vi "saveToTIFF.vi"(1 "Array":i32[][][](array[numeric]), 2 "selected path":path=path "C:/Users/Administrator/Desktop/tiff.tiff") -> ()   [LabVIEW 2016]
panel:
  out "max value 2":u16
  out "max value":u16
  out "Intensity Graph 2":u16[][](graph)
  in  "path to JPEG file":path=path "C:/Users/Administrator/Desktop/tiff.jpeg"
  out "Intensity Graph":u16[][](graph)
  in  "file path (use dialog)":path=path "C:/Users/Administrator/Desktop/binary.txt"
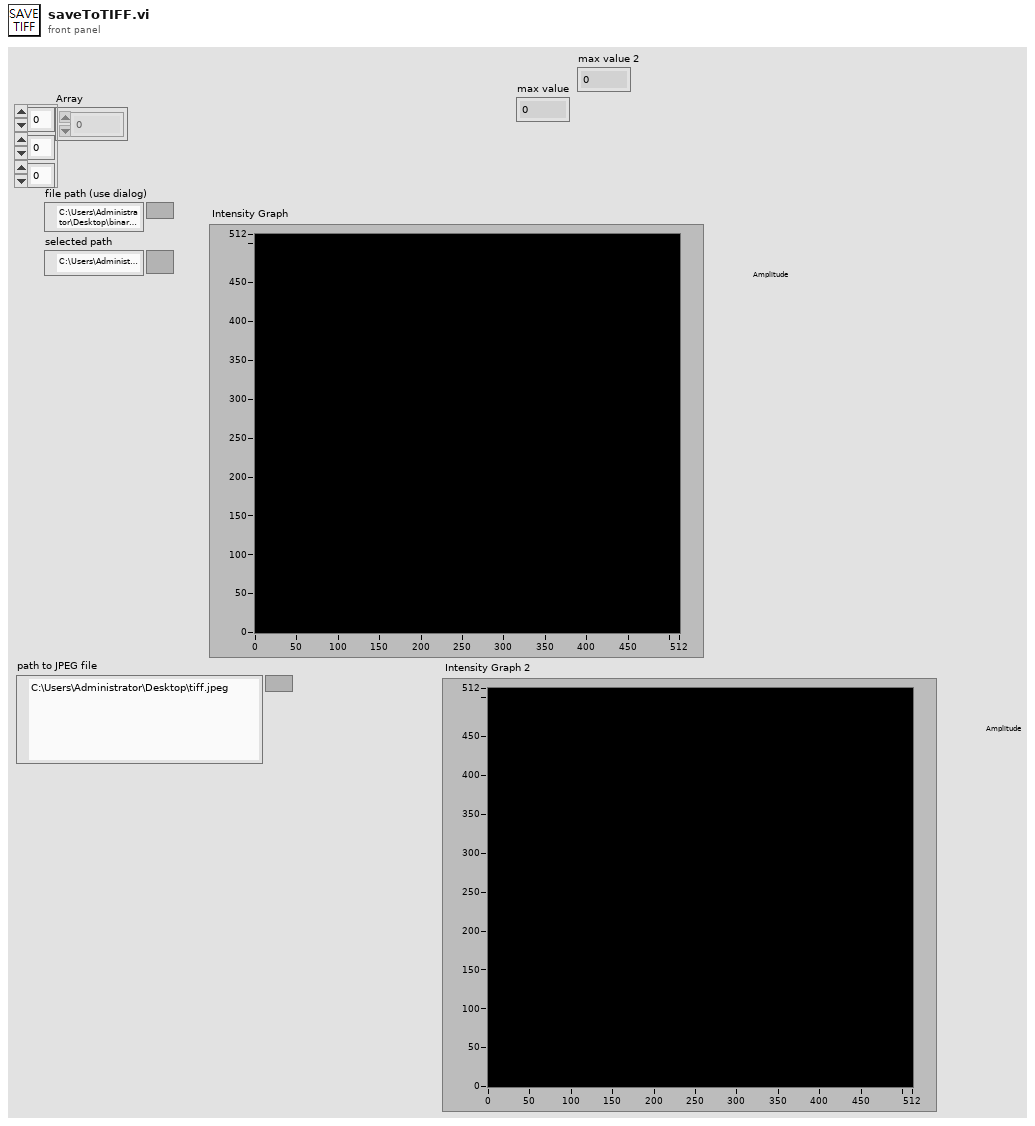
[diagram p1: front panel]
types:
  T1 = cluster{"SPEC":cluster{"CCD":cluster{"ModuleNo":string, "SerialNo":string, "CCD Type":string, "Counts":i32, "PixelNumber":i32, "PixelSize":dbl, "Exposure(ms )":dbl, "Average":i32, "Boxcar":i32, "binFactor":i32, "Reversion":bool, "Andor":cluster{"Temp. Target":i32, "Temp Stablized?":bool, "Readout List":string[], "RreAmp List":string[], "VSS List":string[], "Readout":u16, "PreAmp":u16, "VSS":u16, "Temp. Min":i32, "Temp. Max":i32, "OutputAmp List":string[], "OutputAmp":u16}, "Kinetic No":i32, "AccumCT":dbl, "KineticCT":dbl, "AcqMode":enum16{"Monitor", "Acquisition"}, "SpectraProcess":enum16{"Absorption", "TakeRef", "TakeBG", "Substraction", "Transmission", "ClearRef", "ClearBG", "Default"}, "Real AccumCT":dbl, "Real KineticCT":dbl, "Real Exposure":dbl, "Ref":sgl[], "Graph":cluster{"X ":sgl[], "Y":sgl[]}, "Center to":dbl, "Pulse":dbl, "X Mode":enum16{"Wavelength (nm)", "Pixel (um)", "Raman Shift (cm^-1)"}, "Background":sgl[], "Scan":bool}, "SPEC Name":string, "User":cluster{"COM":string, "GratingNo ":i32, "Interval (ms )":i32, "Laser (nm)":dbl}, "Gratings with PAT":cluster{"Grating Name":string, "Grating Groove":dbl, "Grating Blaze":dbl, "Zero Position":dbl, "Half Turn":dbl, "Focal Length":dbl, "Grating Offset(a0)":dbl, "Detector Offset(a1)":dbl, "Dispersion Angle":dbl, "Center Pixel At":dbl, "Focal Plane Angle":dbl, "Negative Order":bool, "FixSpec":dbl[], "Kcoeff":dbl, "Fcoeff":dbl, "Dcoeff":dbl}[], "ShutterID":i32, "Scanner4":cluster{"Total Frames":i32, "Frames Dwell(s)":dbl, "Z-Stack":bool}, "SPEC Type":string}, "i":u32}
  T2 = enum16{"big-endian, network order", "native, host order", "little-endian"}
  T3 = typedef "imagedata.ctl" = cluster{"image type":i32, "image depth":i32, "image":u8[], "mask":u8[], "colors":u32[], "Rectangle":cluster{"left":i16, "top":i16, "right":i16, "bottom":i16}}
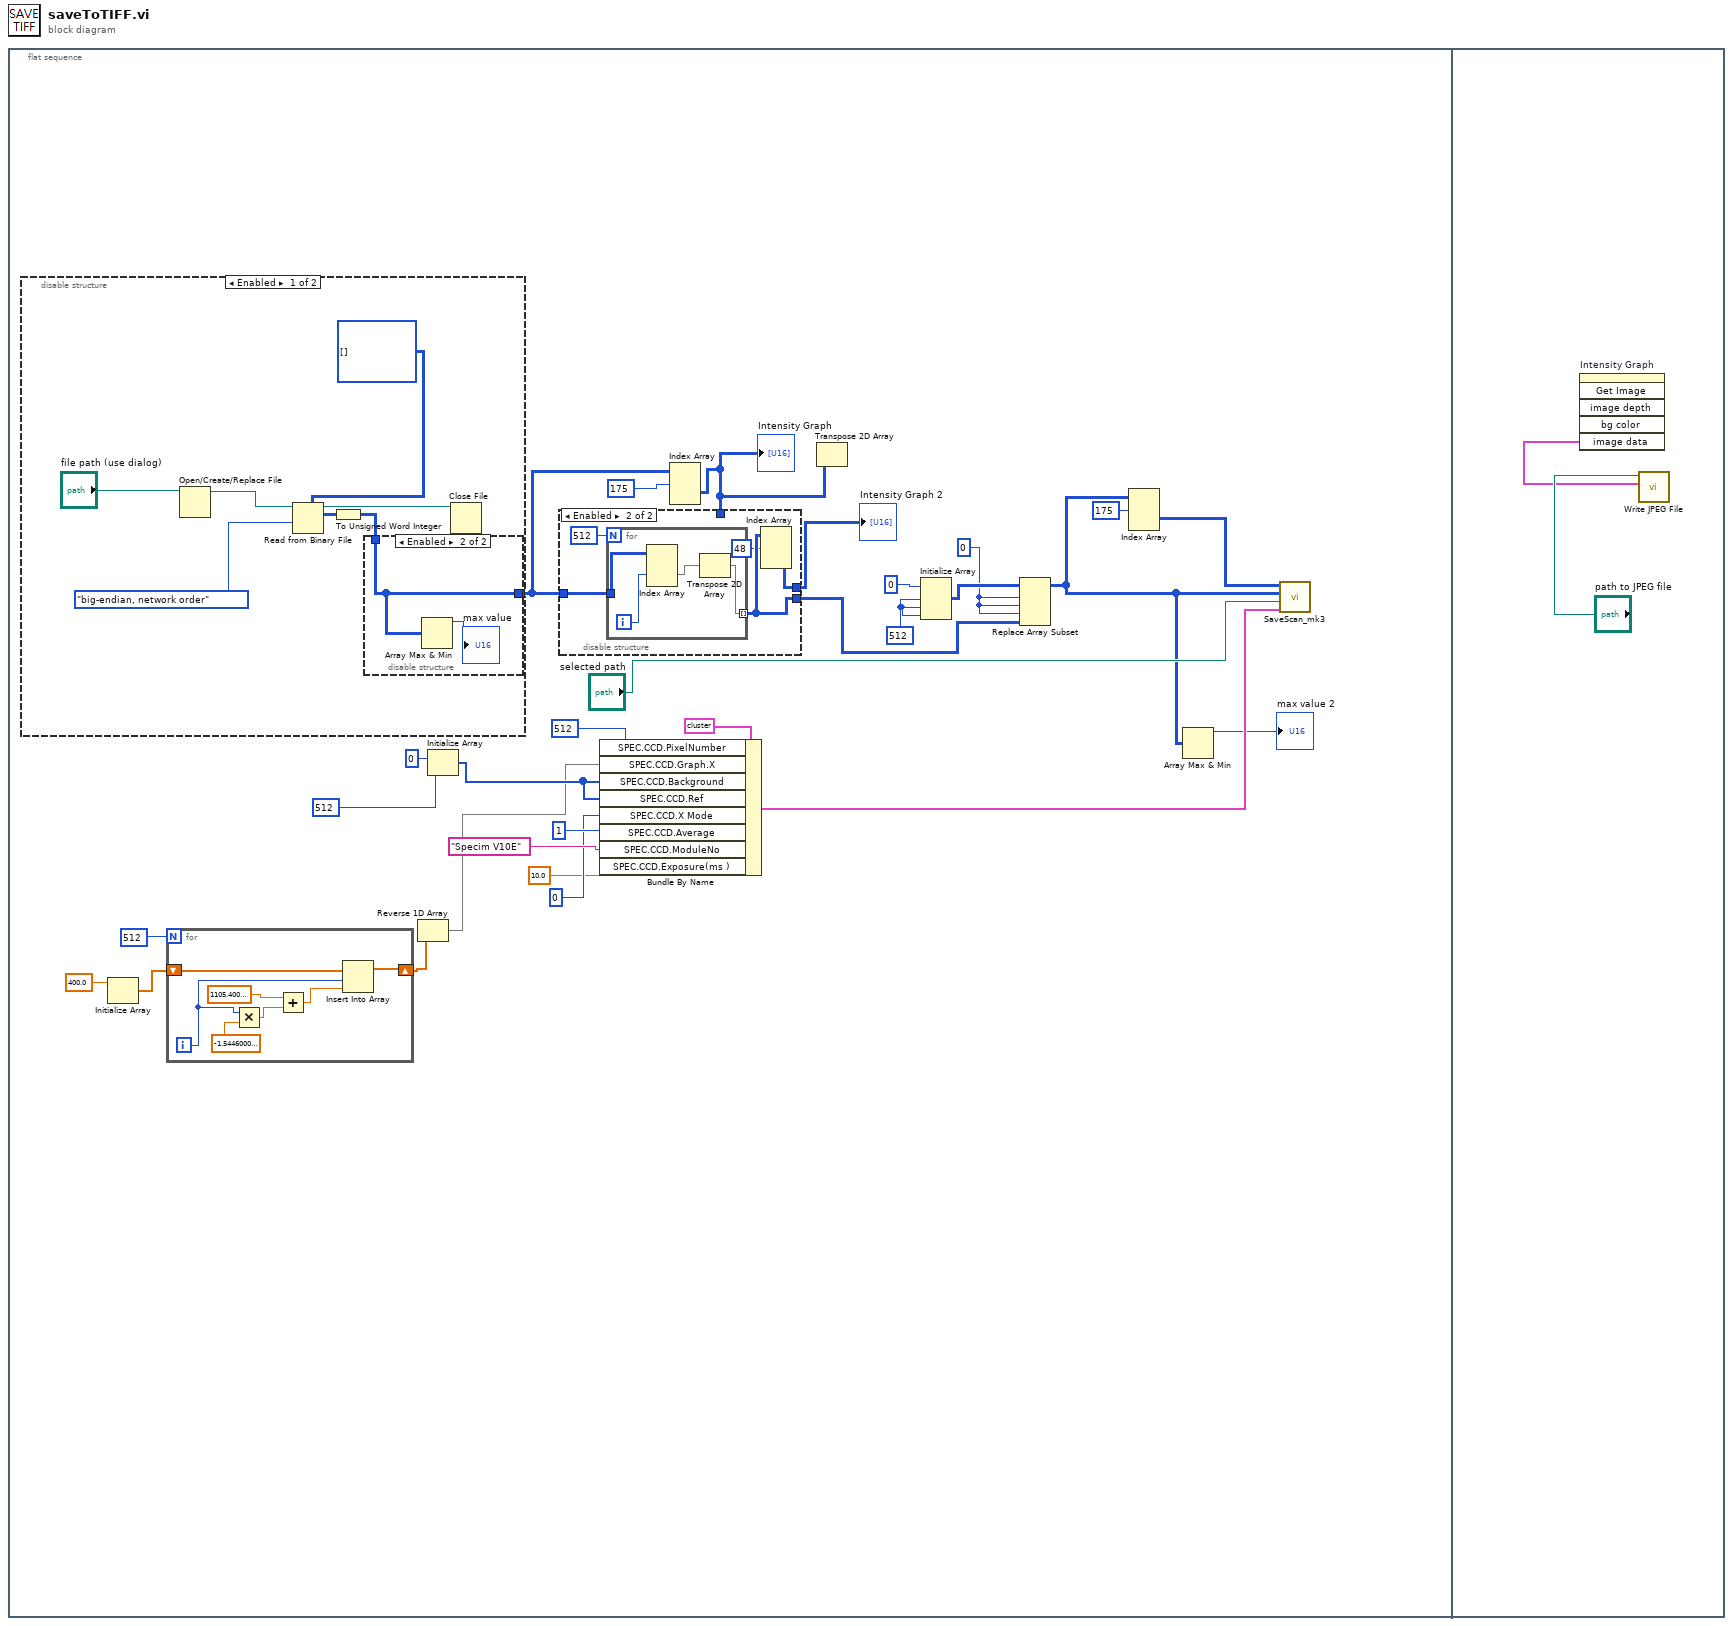
[diagram p0: block diagram]
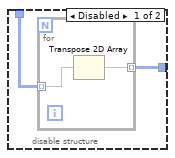
[diagram p2: hidden frame]
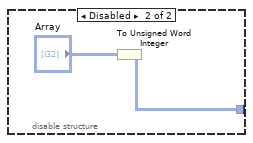
[diagram p3: hidden frame]
diagram:
  n1 = flat-sequence {
    frame #0 {
      w4 = 0 ("index (page)")
      w7 = 512 ("dimension size")
      n2 = disable-structure shown="Enabled" {
        disable-tunnel: [w30 w44] -> w28
        frame Enabled {
          n3 = Open/Create/Replace File(file path (use dialog)="file path (use dialog)") -> (refnum out=w36:refnum<file>)  [unwired: 5 in, 2 out]
          n4 = Read from Binary File(5:i32[][][] [], 9:T2."big-endian, network order" ("byte order (0:big-endian, network order)"), 11:w36) -> (2:w32:i32[][][], 3:w35:refnum<file>)  [unwired: 3 in, 2 out]
          n5 = To Unsigned Word Integer(number=w32) -> (unsigned 16bit integer=w31:u16[][][])
          n6 = disable-structure shown="Enabled" {
            disable-tunnel: w31 -> [w39 w43]
            disable-tunnel: [w38 w43] -> w30
            frame Disabled {
              n7 = for {
                tunnel: w39 -> [w41] mode=indexing
                tunnel: [w40] -> w38 mode=indexing
                n8 = Transpose 2D Array(2D array=w41) -> (transposed array=w40:u16[][])
              }
            }
            frame Enabled {
              n9 = Array Max & Min(array=w43) -> (max value=→"max value":u16)  [unwired: 3 out]
            }
          }
          n10 = Close File(refnum=w35) -> ()  [unwired: 1 in, 2 out]
        }
        frame Disabled {
          n11 = To Unsigned Word Integer(number="Array") -> (unsigned 16bit integer=w44:u16[][][])
        }
      }
      n12 = Initialize Array(sgl 400.0 ("element")) -> (w22:sgl[])  [unwired: 1 in]
      n13 = for {
        N: 512 -> [_]
        shift-right: [w51] -> w21
        shift-left: w22 -> [w52]
        i -> [w50]
        n14 = Multiply(x=w50, y=sgl -1.5446) -> (x*y=w48:sgl)
        n15 = Add(x=sgl 1105.4, y=w48) -> (x+y=w46:sgl)
        n16 = Insert Into Array(array=w52, index=w50, new element=w46) -> (w51:sgl[])
      }
      n17 = Reverse 1D Array(array=w21) -> (reversed array=w14:sgl[])
      n18 = Initialize Array(u16 0 ("element"), 512 ("dimension size")) -> (w15:u16[])
      n19 = Bundle By Name(cluster=T1 {"SPEC"={"CCD"={"ModuleNo"="HIS-Specim", "SerialNo"="V10E", "CCD Type"="iXon", "Counts"=0, "PixelNumber"=512, "PixelSize"=0.0, "Exposure(ms )"=0.0, "Average"=0, "Boxcar"=0, "binFactor"=1, "Reversion"=FALSE, "Andor"={"Temp. Target"=0, "Temp Stablized?"=FALSE, "Readout List"=[], "RreAmp List"=[], "VSS List"=[], "Readout"=0, "PreAmp"=0, "VSS"=0, "Temp. Min"=0, "Temp. Max"=0, "OutputAmp List"=[], "OutputAmp"=0}, "Kinetic No"=0, "AccumCT"=0.0, "KineticCT"=0.0, "AcqMode"=enum."Monitor", "SpectraProcess"=enum."Default", "Real AccumCT"=0.0, "Real KineticCT"=0.0, "Real Exposure"=0.0, "Ref"=[], "Graph"={"X "=[], "Y"=[]}, "Center to"=0.0, "Pulse"=0.0, "X Mode"=enum."Wavelength (nm)", "Background"=[], "Scan"=FALSE}, "SPEC Name"="", "User"={"COM"="", "GratingNo "=0, "Interval (ms )"=0, "Laser (nm)"=0.0}, "Gratings with PAT"=[], "ShutterID"=0, "Scanner4"={"Total Frames"=0, "Frames Dwell(s)"=0.0, "Z-Stack"=FALSE}, "SPEC Type"=""}, "i"=0} ("Spec metadata"), "SPEC.CCD.PixelNumber"=512, "SPEC.CCD.Graph.X"=w14, "SPEC.CCD.Background"=w15, "SPEC.CCD.Ref"=w15, "SPEC.CCD.X Mode"=u8 0, "SPEC.CCD.Average"=u8 1, "SPEC.CCD.ModuleNo"="Specim V10E", "SPEC.CCD.Exposure(ms )"=sgl 10.0) -> (w26:T1)
      n20 = Index Array(array=w28, index (dim 0)=175 ("index (page)")) -> (element=w18:u16[][])  [unwired: 2 in]
      "Intensity Graph" <- w18
      n21 = disable-structure shown="Enabled" {
        disable-tunnel: [w54 w58] -> w20
        disable-tunnel: w18 -> [w54 _]
        disable-tunnel: [w53 w59] -> w5
        disable-tunnel: w28 -> [w53 w56]
        frame Disabled {
        }
        frame Enabled {
          n22 = for {
            N: 512 -> [_]
            tunnel: w56 -> [w63]
            tunnel: [w62] -> w59 mode=indexing
            i -> [w60]
            n23 = Index Array(array=w63, index (dim 1)=w60) -> (element=w61:u16[][])  [unwired: 2 in]
            n24 = Transpose 2D Array(2D array=w61) -> (transposed array=w62:u16[][])
          }
          n25 = Index Array(array=w59, index (dim 0)=48 ("index (page)")) -> (element=w58:u16[][])  [unwired: 2 in]
        }
      }
      "Intensity Graph 2" <- w20
      n26 = Transpose 2D Array(2D array=w18) -> ()  [unwired: 1 out]
      n27 = Initialize Array(u16 0 ("element"), w7, w7, w7) -> (w6:u16[][][])
      n28 = Replace Array Subset(array=w6, new element=w5, index (dim 0)=w4, index (dim 1)=w4, index (dim 2)=w4) -> (w1:u16[][][])
      n29 = Index Array(array=w1, index (dim 0)=175 ("index (page)")) -> (element=w2:u16[][])  [unwired: 2 in]
      n30 = Array Max & Min(array=w1) -> (max value=→"max value 2":u16)  [unwired: 3 out]
      n31 = call "SaveScan_mk3.vi"("Display Array"=w2, "Array"=w1, "selected path"="selected path", "Spec metadata"=w26) -> ()  [unwired: 7 in]
    }
    frame #1 {
      n32 = invoke on="Intensity Graph" class="IntGraph (strict)" method="Get Image"() -> ("image data"=w64:T3)  [unwired: 6 in, 5 out]
      n33 = call <vilib>:"Write JPEG File.vi"("image data"=w64, "path to JPEG file"="path to JPEG file") -> ()  [unwired: 8 in, 2 out]
    }
  }
